vi "DropTableDbUnderstanding.vi"() -> ()   [LabVIEW 2019]
uses:
  <vilib>/addons/database/Connection.llb/DB Tools Open Connec (String).vi
  <vilib>/addons/database/NI_Database_API.lvlib
panel:
  in  "Enter the Table Name which you want to delete":string
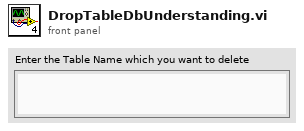
[diagram p1: front panel]
types:
  T1 = typedef "NI_Database_API.lvlib/Conn ObjectReference.ctl" = refnum<k1>
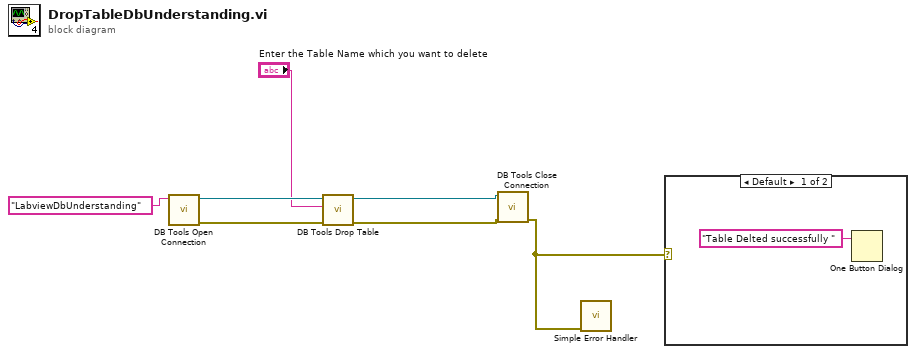
[diagram p0: block diagram]
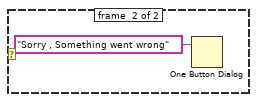
[diagram p2: hidden frame]
diagram:
  n1 = call-poly <vilib>:"DB Tools Open Connection.vi"("connection information"="LabviewDbUnderstanding") -> ("error out"=w7:errorcluster, "connection reference"=w6:T1)  [unwired: 7 in]
  n2 = call <vilib>:"DB Tools Drop Table.vi"("error in (no error)"=w7, "table"="Enter the Table Name which you want to delete", "connection reference"=w6) -> ("error out"=w4:errorcluster, "connection reference out"=w5:T1)  [unwired: 5 in]
  n3 = call <vilib>:"DB Tools Close Connection.vi"("error in (no error)"=w4, "connection reference"=w5) -> ("error out"=w1:errorcluster)  [unwired: 5 in]
  n4 = call <vilib>:"Simple Error Handler.vi"("error in (no error)"=w1) -> ()  [unwired: 4 in, 5 out]
  n5 = case shown="Default" w1 {
    frame #0 {
      n6 = One Button Dialog(message="Table Delted successfully ") -> ()  [unwired: 1 in, 1 out]
    }
    frame #1 {
      n7 = One Button Dialog(message="Sorry , Something went wrong") -> ()  [unwired: 1 in, 1 out]
    }
  }
